vi "Get FPGA Dependent File.vi"(8 "error in (no error)":errorcluster, 11 "ID in":T1 format="%.0x") -> (0 "error out":errorcluster, 2 "RT Path":path, 3 "ID out":T1 format="%.0x")   [LabVIEW 2015, in "AIT 429 System Explorer.lvlib"]
uses:
  <vilib>/NI Veristand/Custom Device API/Custom Device Item Ref.ctl
  NationalInstruments.VeriStand.SystemDefinitionAPI
  AIT 429 System Explorer.lvlib
  <vilib>/NI Veristand/Custom Device Offline API/Custom Device Offline API.lvlib
  <vilib>/NI Veristand/Custom Device API/Custom Device API.lvlib
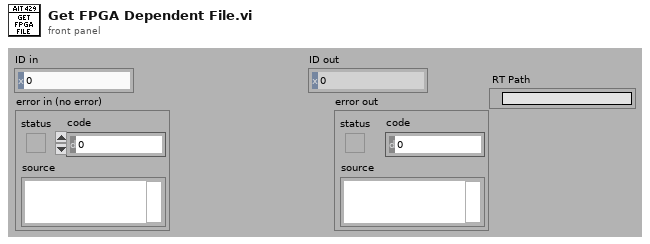
[diagram p1: front panel]
types:
  T1 = typedef "Custom Device API.lvlib/Custom Device Item Ref.ctl" = u64
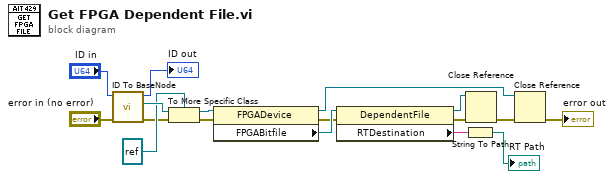
[diagram p0: block diagram]
diagram:
  n1 = call <vilib>:"ID To BaseNode.vi"("error in (no error)"="error in (no error)", "ID in"="ID in") -> ("error out"=w15:errorcluster, "BaseNode"=w17:refnum<k24>, "ID out"=→"ID out":u64)  [unwired: 7 in]
  n2 = To More Specific Class(target class=refnum<k24> refnum ("BaseNodeType"), reference=w17, error in=w15) -> (specific class reference=w14:refnum<k24>, error out=w13:errorcluster)
  n3 = property class="FPGADevice"(reference=w14, error in=w13) -> (reference out=w8:refnum<k24>, error out=w6:errorcluster, "FPGABitfile"=w7:refnum<k24>)
  n4 = property class="DependentFile"(reference=w7, error in=w6) -> (reference out=w4:refnum<k24>, error out=w5:errorcluster, "RTDestination"=w2:string)
  n5 = String To Path(string=w2) -> (path=→"RT Path":path)
  n6 = Close Reference(reference=w4, error in (no error)=w5) -> (error out=w3:errorcluster)
  n7 = Close Reference(reference=w8, error in (no error)=w3) -> (error out=→"error out":errorcluster)
